vi "ArmGlobal.vi"() -> ()   [LabVIEW 2020]
doc: "Global varables for Arm"
panel:
  out "ArmUpDown":bool
  out "TargetGamePiece":string
  out "TargetSideRobot":string
  out "TargetArmPosition":string
  out "RotateOnTarget":bool
  out "RLEOnTarget":bool
  out "LiftOnTarget":bool
  out "ExtendOnTarget":bool
  out "ZPosition":dbl
  out "YPosition":dbl
  out "XPosition":dbl
  out "ZDemand":dbl
  out "YDemand":dbl
  out "XDemand":dbl
  out "ExtendPostion":dbl
  out "LiftPostion":dbl
  out "RotatePostion":dbl
  out "ExtendMotorOutput":dbl
  out "LiftMotorOutput":dbl
  out "RotateMotorOutput":dbl
  out "RotatePositonDemand(d)":dbl
  out "ExtendPositonDemand(in)":dbl
  out "LiftPositionDemand(d)":dbl
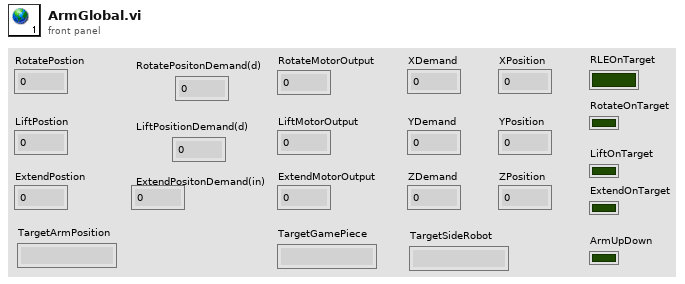
[diagram p1: front panel]
diagram:
